vi "ButtonState.vi"(8 "error in (no error)":errorcluster, 11 "Button in":refnum<class "Button.lvclass">) -> (0 "error out":errorcluster, 3 "Button out":refnum<class "Button.lvclass">)   [LabVIEW 2019, in "Button.lvclass"]
doc: "Uses RefNum to extract IP Address. Then uses TCP Open/Close on Port 80 with a 2sec timeout to see if the button is ON and then updates the Boolean value on the Front Panel and it's value in the Object private data."
uses:
  Button.lvclass
  Button.lvclass/Button.ctl
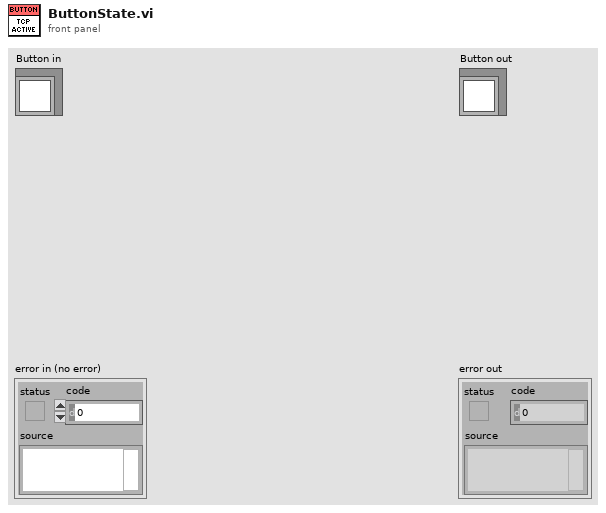
[diagram p1: front panel]
types:
  T1 = enum16{"Standard", "Buffered", "CRLF", "Immediate"}
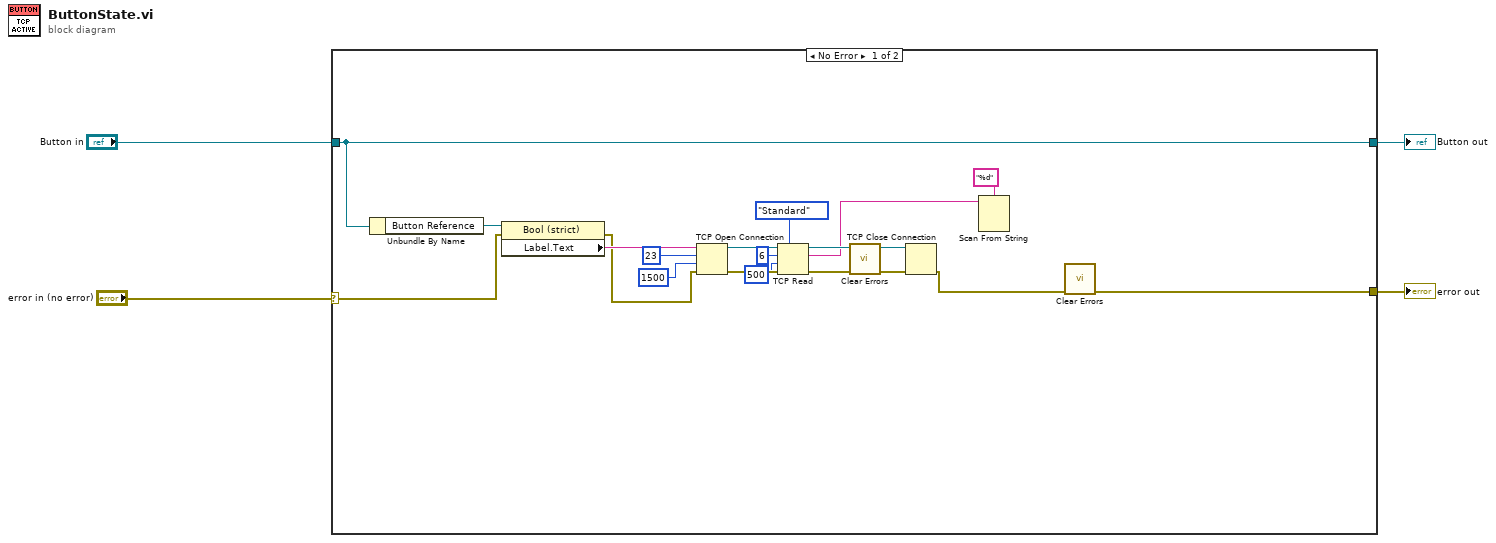
[diagram p0: block diagram]
diagram:
  n1 = case shown="No Error" "error in (no error)" {
    selector: "error in (no error)" -> [w18 w25]
    tunnel: [w6 w25] -> w4
    tunnel: [w20 w24] -> w3
    tunnel: "Button in" -> [w20 w24]
    frame No Error {
      n2 = Unbundle By Name(w20) -> ("Button Reference"=w23:refnum<vi>)
      n3 = property class="Bool (strict)"(reference=w23, error in=w18) -> (error out=w19:errorcluster, "Label.Text"=w22:string)  [unwired: 1 out]
      n4 = TCP Open Connection(address=w22, remote port or service name=u16 23, timeout ms (60000)=1500, error in (no error)=w19) -> (connection ID=w17:refnum<k5>, error out=w15:errorcluster)  [unwired: 1 in]
      n5 = TCP Read(connection ID=w17, bytes to read=6, error in (no error)=w15, 7:T1."Standard" ("mode (standard)"), 9:500 ("timeout ms (25000)")) -> (connection ID out=w16:refnum<k5>, data out=w8:string, error out=w11:errorcluster)
      n6 = call <vilib>:"Clear Errors.vi"("error in (no error)"=w11) -> ("error out"=w10:errorcluster)  [unwired: 5 in, 1 out]
      n7 = TCP Close Connection(connection ID=w16, error in (no error)=w10) -> (error out=w7:errorcluster)  [unwired: 1 in, 1 out]
      n8 = Scan From String(format string="%d", input string=w8) -> ()  [unwired: 4 in, 3 out]
      n9 = call <vilib>:"Clear Errors.vi"("error in (no error)"=w7) -> ("error out"=w6:errorcluster)  [unwired: 5 in, 1 out]
    }
    frame Error {
    }
  }
  "error out" <- w4
  "Button out" <- w3
